vi "niRFUtil MEAS Frequency Offset (Hz).vi"(0 "Waveform In":T4 {"y" format="%.2f"; "dx" format="%^.2e"; "x0" format="%^.2e"}, 1 "Apply Frequency Offset":T1, 5 "Reference Waveform In":T4 {"y" format="%.2f"; "dx" format="%^.2e"; "x0" format="%^.2e"}, 7 "Filter Phase Estimates":T3=enum."True", 9 "Filter Length (samples)":i32=20, 11 "Iterations":i32=2, 12 "DC Offset Correction":T2=enum."True", 13 "Origin Offset Threshold (dBm)":sgl=inf) -> (3 "Gain (dB)":sgl, 4 "Waveform Out":T4 {"y" format="%.2f"; "dx" format="%^.2e"; "x0" format="%^.2e"}, 6 "Reference Waveform Out":T4 {"y" format="%.2f"; "dx" format="%^.2e"; "x0" format="%^.2e"}, 8 "Frequency Offset (Hz)":sgl format="%^.2e", 10 "Phase Offset (deg)":sgl format="%.2f", 15 "Origin Offset":csg format="%.4f")   [LabVIEW 2015, in "niRFUtil.lvlib"]
uses:
  niRFUtil.lvlib
  Includes/niRFUtil INC Complex Waveform.ctl
  Includes/niRFUtil INC Complex Array.ctl
  Includes/niRFUtil INC Filter Phase Estimates.ctl
  Includes/niRFUtil INC Origin Offset Correction.ctl
  Includes/niRFUtil INC Apply Frequency Offset.ctl
  Waveform Manipulation/niRFUtil WFM Apply Linear Gain (complex wfm).vi
  Waveform Manipulation/niRFUtil WFM Moving Average (complex array).vi
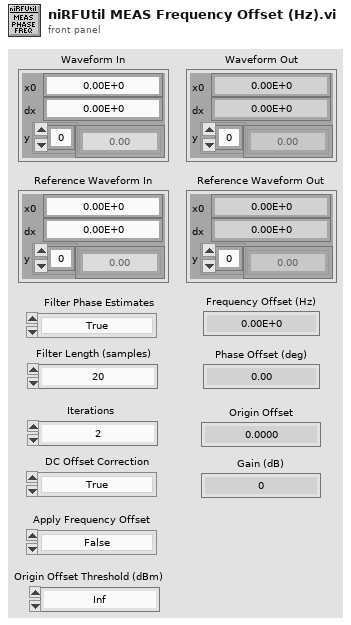
[diagram p1: front panel]
types:
  T1 = typedef "niRFUtil.lvlib/niRFUtil INC Apply Frequency Offset.ctl" = enum16{"False", "True"}
  T2 = typedef "niRFUtil.lvlib/niRFUtil INC Origin Offset Correction.ctl" = enum16{"False", "True"}
  T3 = typedef "niRFUtil.lvlib/niRFUtil INC Filter Phase Estimates.ctl" = enum16{"False", "True"}
  T4 = typedef "niRFUtil.lvlib/niRFUtil INC Complex Waveform.ctl" = cluster{"x0":dbl, "dx":dbl, "y":T5}
  T5 = typedef "niRFUtil.lvlib/niRFUtil INC Complex Array.ctl" = csg[]
  T6 = typedef "niRFUtil.lvlib/niRFUtil INC Real Array.ctl" = sgl[]
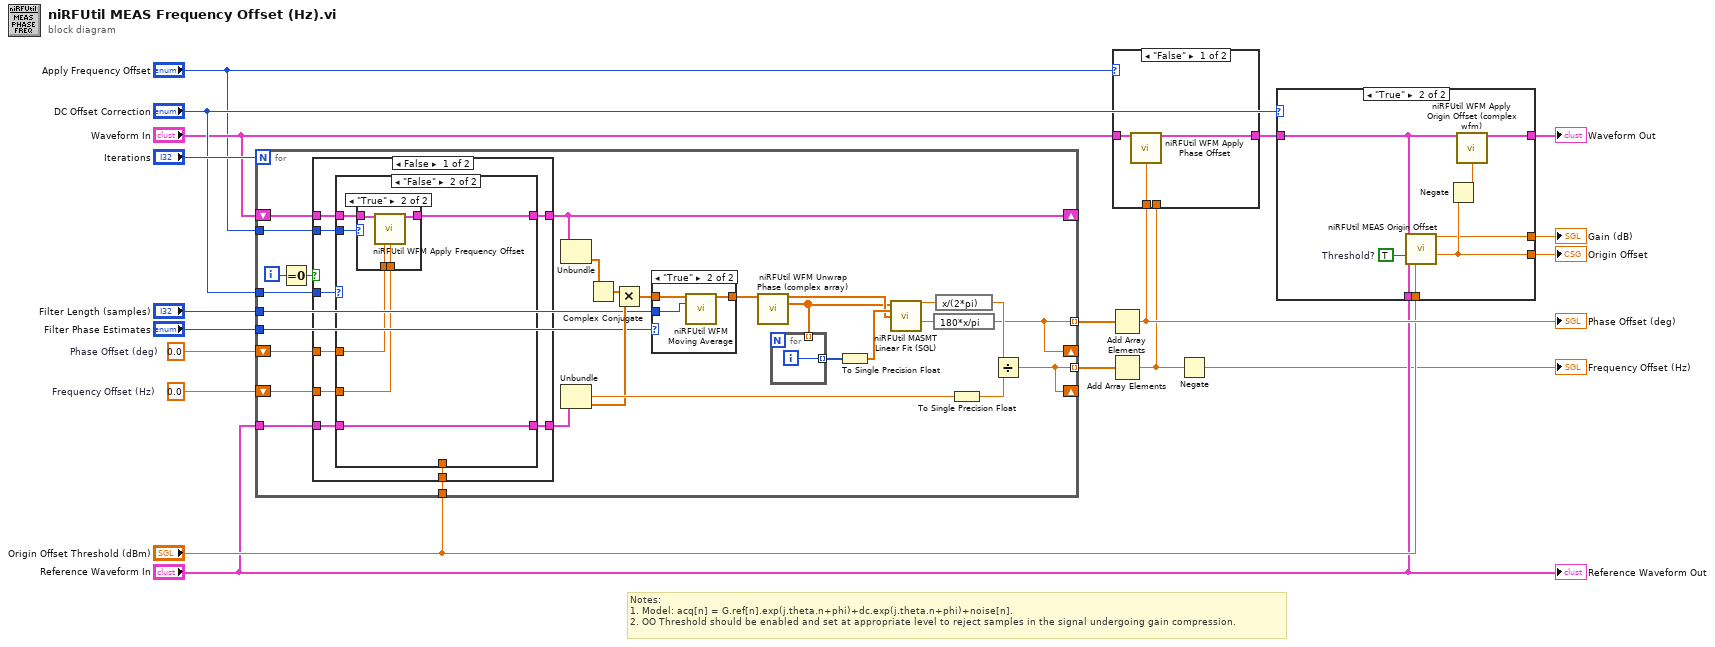
[diagram p0: block diagram]
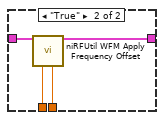
[diagram p2: hidden frame]
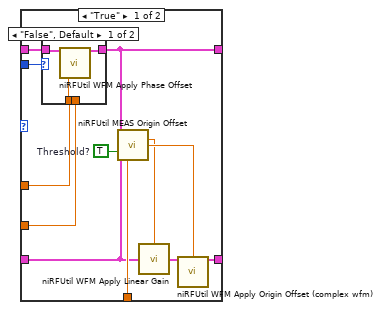
[diagram p3: hidden frame]
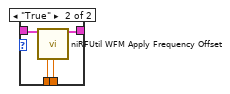
[diagram p4: hidden frame]
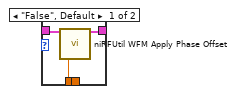
[diagram p5: hidden frame]
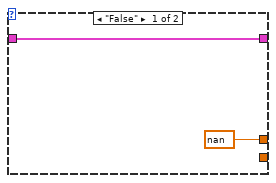
[diagram p8: hidden frame]
diagram:
  w14 = sgl 0.0  # Phase Offset (deg)
  w15 = sgl 0.0  # Frequency Offset (Hz)
  # "Notes:\n1. Model: acq[n] = G.ref[n].exp(j.theta.n+phi)+dc.exp(j.theta.n+phi)+noise[n].\n2. OO Threshold should be enabled and set at appropriate level to reject samples in the signal undergoing gain compression."
  n1 = for {
    N: "Iterations" -> [_]
    tunnel: [w21] -> w2 mode=indexing
    tunnel: [w32] -> w16 mode=indexing
    tunnel: "Filter Phase Estimates" -> [w37]
    tunnel: "Filter Length (samples)" -> [w36]
    shift-right: [w28] -> _
    shift-left: "Waveform In" -> [w34]
    shift-right: [w21] -> _
    shift-left: w15 -> [w27]
    shift-right: [w32] -> _
    shift-left: w14 -> [w31]
    tunnel: "DC Offset Correction" -> [w29]
    tunnel: "Origin Offset Threshold (dBm)" -> [w23]
    tunnel: "Reference Waveform In" -> [w24]
    tunnel: "Apply Frequency Offset" -> [w20]
    i -> [w33]
    n2 = Equal To 0?(x=w33) -> (x = 0?=w26:bool)
    n3 = case shown="False" w26 {
      tunnel: [w57 w91] -> w28
      tunnel: w34 -> [w53 w91]
      tunnel: w24 -> [w56 w90]
      tunnel: w31 -> [w54 _]
      tunnel: w27 -> [w55 _]
      tunnel: w29 -> [w49 _]
      tunnel: w23 -> [w52 _]
      tunnel: [w51 w90] -> w22
      tunnel: w20 -> [w50 _]
      frame False {
        n4 = case shown="\"False\"" w49 {
          tunnel: [w67 w80] -> w57
          tunnel: w56 -> [w64 w82]
          tunnel: w55 -> [w61 w78]
          tunnel: w54 -> [w68 w79]
          tunnel: w53 -> [w69 w81]
          tunnel: w52 -> [w65 _]
          tunnel: [w63 w82] -> w51
          tunnel: w50 -> [w58 w77]
          frame "True" {
            w66 = TRUE  # Threshold?
            n5 = case shown="\"False\", Default" w58 {
              tunnel: w69 -> [w72 w76]
              tunnel: w68 -> [w70 w75]
              tunnel: [w71 w74] -> w67
              tunnel: w61 -> [_ w73]
              frame "False", Default {
                n6 = call "niRFUtil WFM Apply Phase Offset.vi"("Waveform In"=w72, "Offset, degrees"=w70) -> ("Waveform Out"=w71:T4)  [unwired: 13 in]
              }
              frame "True" {
                n7 = call "niRFUtil WFM Apply Frequency Offset.vi"("Waveform In"=w76, "Initial Phase (deg)"=w75, "Offset (Hz)"=w73) -> ("Waveform Out"=w74:T4)  [unwired: 11 in, 1 out]
              }
            }
            n8 = call "niRFUtil MEAS Origin Offset.vi"("Waveform In"=w67, "Reference Waveform In"=w64, "Threshold?"=w66, "Origin Offset Threshold (dBm)"=w65) -> ("Gain (linear)"=w59:sgl, "Origin Offset"=w62:csg)  [unwired: 8 in, 2 out]
            n9 = call-poly "niRFUtil WFM Apply Linear Gain.vi"("Gain"=w59, "Waveform In"=w64) -> ("Waveform Out"=w60:T4)  [unwired: 2 in]
            n10 = call "niRFUtil WFM Apply Origin Offset (complex wfm).vi"("Waveform In"=w60, "Origin Offset"=w62) -> ("Waveform Out"=w63:T4)  [unwired: 13 in]
          }
          frame "False" {
            n11 = case shown="\"True\"" w77 {
              tunnel: w81 -> [w85 w89]
              tunnel: w79 -> [w83 w88]
              tunnel: [w84 w87] -> w80
              tunnel: w78 -> [_ w86]
              frame "False", Default {
                n12 = call "niRFUtil WFM Apply Phase Offset.vi"("Waveform In"=w85, "Offset, degrees"=w83) -> ("Waveform Out"=w84:T4)  [unwired: 13 in]
              }
              frame "True" {
                n13 = call "niRFUtil WFM Apply Frequency Offset.vi"("Waveform In"=w89, "Initial Phase (deg)"=w88, "Offset (Hz)"=w86) -> ("Waveform Out"=w87:T4)  [unwired: 11 in, 1 out]
              }
            }
          }
        }
      }
      frame True {
      }
    }
    n14 = Unbundle(w28) -> ("y"=w45:T5)  [unwired: 2 out]
    n15 = Unbundle(w22) -> ("dx"=w47:dbl, "y"=w42:T5)  [unwired: 1 out]
    n16 = Complex Conjugate(1:w45) -> (0:w48:T5)
    n17 = Multiply(x=w48, y=w42) -> (x*y=w41:T5)
    n18 = case shown="\"True\"" w37 {
      tunnel: w41 -> [w92 w95]
      tunnel: [w92 w94] -> w40
      tunnel: w36 -> [_ w93]
      frame "False" {
      }
      frame "True" {
        n19 = call-poly "niRFUtil WFM Moving Average.vi"("Array In"=w95, "Averaging Window (samples)"=w93) -> ("Averaged Array Out"=w94:T5)  [unwired: 13 in]
      }
    }
    n20 = call "niRFUtil WFM Unwrap Phase (complex array).vi"("Complex Vectors"=w40) -> ("Magnitude"=w39:T6, "Unwrapped Phase (rad)"=w38:T6)  [unwired: 13 in]
    n21 = for {
      tunnel: [w96] -> w44 mode=indexing
      tunnel: w38 -> [_] mode=indexing
      i -> [w96]
    }
    n22 = To Single Precision Float(number=w44) -> (single precision float=w43:sgl[])
    n23 = call "niRFUtil MASMT Linear Fit (SGL).vi"("Y"=w38, "X"=w43, "Weight"=w39) -> ("slope"=w25:sgl, "intercept"=w30:sgl)  [unwired: 8 in, 3 out]
    n24 = expression code="180*x/pi"(w30) -> (w32:sgl)
    n25 = expression code="x/(2*pi)"(w25) -> (w46:sgl)
    n26 = To Single Precision Float(number=w47) -> (single precision float=w35:sgl)
    n27 = Divide(x=w46, y=w35) -> (x/y=w21:sgl)
  }
  n28 = Add Array Elements(numeric array=w16) -> (sum=w11:sgl)
  "Phase Offset (deg)" <- w11
  n29 = Add Array Elements(numeric array=w2) -> (sum=w10:sgl)
  n30 = case shown="\"False\"" "Apply Frequency Offset" {
    tunnel: "Waveform In" -> [w98 w103]
    tunnel: [w97 w102] -> w5
    tunnel: w11 -> [w99 w101]
    tunnel: w10 -> [_ w100]
    frame "False" {
      n31 = call "niRFUtil WFM Apply Phase Offset.vi"("Waveform In"=w98, "Offset, degrees"=w99) -> ("Waveform Out"=w97:T4)  [unwired: 13 in]
    }
    frame "True" {
      n32 = call "niRFUtil WFM Apply Frequency Offset.vi"("Waveform In"=w103, "Initial Phase (deg)"=w101, "Offset (Hz)"=w100) -> ("Waveform Out"=w102:T4)  [unwired: 11 in, 1 out]
    }
  }
  n33 = Negate(x=w10) -> (-x=→"Frequency Offset (Hz)":sgl)
  n34 = case shown="\"True\"" "DC Offset Correction" {
    tunnel: w5 -> [w105 w110]
    tunnel: [w105 w109] -> w4
    tunnel: "Reference Waveform In" -> [_ w113]
    tunnel: [_ w111] -> w13
    tunnel: "Origin Offset Threshold (dBm)" -> [_ w108]
    tunnel: [sgl nan ("Gain (dB)") w107] -> w8
    frame "False" {
    }
    frame "True" {
      w106 = TRUE  # Threshold?
      n35 = call "niRFUtil MEAS Origin Offset.vi"("Waveform In"=w110, "Reference Waveform In"=w113, "Threshold?"=w106, "Origin Offset Threshold (dBm)"=w108) -> ("Gain (dB)"=w107:sgl, "Origin Offset"=w111:csg)  [unwired: 8 in, 2 out]
      n36 = Negate(x=w111) -> (-x=w112:csg)
      n37 = call "niRFUtil WFM Apply Origin Offset (complex wfm).vi"("Waveform In"=w110, "Origin Offset"=w112) -> ("Waveform Out"=w109:T4)  [unwired: 13 in]
    }
  }
  "Waveform Out" <- w4
  "Origin Offset" <- w13
  "Gain (dB)" <- w8
  "Reference Waveform Out" <- "Reference Waveform In"
